vi "Single pass per array.vi"(10 "Color Box":u32(colorbox), 11 "index":i32) -> (3 "Raw Data":u8[](array[numeric]))   [LabVIEW 2019, in "LED Matrix Host.lvlib"]
uses:
  LED Matrix Host.lvlib
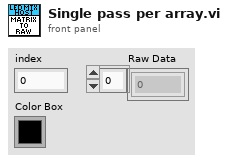
[diagram p1: front panel]
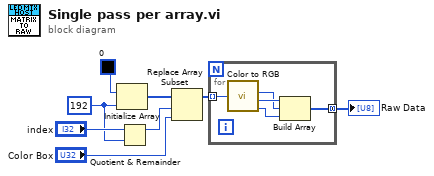
[diagram p0: block diagram]
diagram:
  w2 = 192 ("dimension size")
  n1 = Initialize Array(u32 0, w2) -> (w6:u32[])
  n2 = Quotient & Remainder(x="index", y=w2) -> (x-y*floor(x/y)=w1:i32)  [unwired: 1 out]
  n3 = Replace Array Subset(array=w6, new element="Color Box", index=w1) -> (w4:u32[])
  n4 = for {
    tunnel: w4 -> [w13] mode=indexing
    tunnel: [w9] -> w8 mode=concatenating
    n5 = call <vilib>:"Color to RGB.vi"("Color"=w13) -> ("R"=w11:u8, "G"=w12:u8, "B"=w10:u8)  [unwired: 1 out]
    n6 = Build Array(w12, w11, w10) -> (w9:u8[])
  }
  "Raw Data" <- w8
